vi "Untitled 6 (SubVI).vi"(10 "Numeric 2":i32, 11 "Numeric":dbl) -> (3 "Boolean":bool)   [LabVIEW 2015]
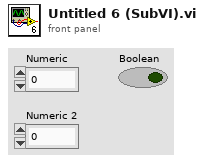
[diagram p1: front panel]
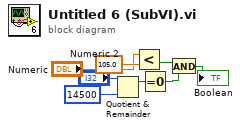
[diagram p0: block diagram]
diagram:
  n1 = Quotient & Remainder(x="Numeric 2", y=14500) -> (x-y*floor(x/y)=w2:i32)  [unwired: 1 out]
  n2 = Less?(x="Numeric", y=105.0) -> (x < y?=w6:bool)
  n3 = Equal To 0?(x=w2) -> (x = 0?=w7:bool)
  n4 = And(x=w6, y=w7) -> (x .and. y?=→"Boolean":bool)
